vi "FPGA Personality.vi"   [LabVIEW 2020]
uses:
  <vilib>/rvi/Emulation/niFpgaGetClockAttributes.vi
  <vilib>/rvi/Emulation/niFpgaSctlEmulationGetInTimedLoop.vi
  <vilib>/rvi/Emulation/niFpgaEmulationReportErrorSimple.vi
  <vilib>/rvi/Emulation/niFpgaCriticalErrorInLSC.vi
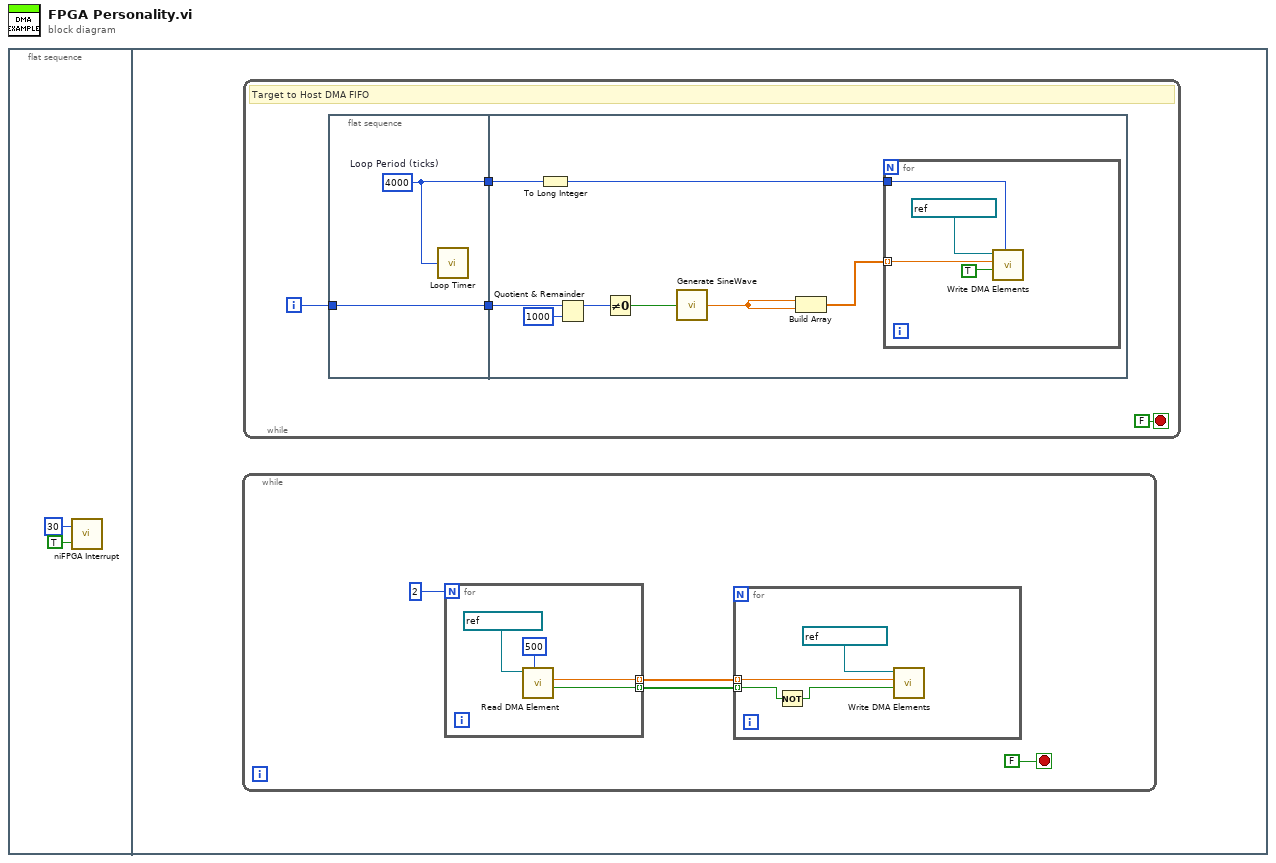
[diagram p0: block diagram]
diagram:
  n1 = flat-sequence {
    frame #0 {
      n2 = call <vilib>:"niFPGA Interrupt.vi"("Wait Until Cleared (F)"=TRUE, "IRQ Number (0)"=u8 30) -> ()  [unwired: 1 in]
    }
    frame #1 {
      n3 = while {
        stop <- FALSE stop-if-true
        n4 = for {
          N: 2 -> [_]
          tunnel: [w12] -> w4 mode=indexing
          tunnel: [w11] -> w3 mode=indexing
          n5 = call "Read DMA Element.vi"("Timeout"=500, "DMA Refnum in"=refnum<k21> "Incoming" ("FIFO In")) -> ("isTimeout ?"=w11:bool, "DMA Element"=w12:sgl)  [unwired: 7 in, 1 out]
        }
        n6 = for {
          tunnel: w4 -> [w8] mode=indexing
          tunnel: w3 -> [w7] mode=indexing
          n7 = Not(x=w7) -> (.not. x?=w9:bool)
          n8 = call "Write DMA Elements.vi"("isValid ?"=w9, "DMA Element"=w8, "FIFO Refnum in"=refnum<k21> "Outgoing2" ("FIFO In")) -> ()  [unwired: 8 in, 1 out]
        }
      }
      n9 = while {
        i -> [w16]
        stop <- FALSE stop-if-true
        # "Target to Host DMA FIFO"
        n10 = flat-sequence {
          tunnel: [w20] -> w18
          tunnel: w16 -> [w19]
          tunnel: [w19] -> w15
          tunnel: w18 -> [w28]
          tunnel: w15 -> [w24]
          frame #0 {
            w20 = u32 4000  # Loop Period (ticks)
            n11 = call "Loop Timer"("Count(Ticks)"=w20) -> ()  [unwired: 1 out]
          }
          frame #1 {
            n12 = To Long Integer(number=w28) -> (32bit integer=w27:i32)
            n13 = Quotient & Remainder(x=w24, y=1000) -> (x-y*floor(x/y)=w22:i32)  [unwired: 1 out]
            n14 = Not Equal To 0?(x=w22) -> (x != 0?=w21:bool)
            n15 = call "Generate SineWave.vi"("GenSine"=w21) -> ("Sine Point"=w25:sgl)
            n16 = Build Array(w25, w25) -> (w26:sgl[])
            n17 = for {
              tunnel: w27 -> [w30]
              tunnel: w26 -> [w29] mode=indexing
              n18 = call "Write DMA Elements.vi"("Timeout"=w30, "isValid ?"=TRUE, "DMA Element"=w29, "FIFO Refnum in"=refnum<k21> "Outgoing1" ("FIFO In")) -> ()  [unwired: 7 in, 1 out]
            }
          }
        }
      }
    }
  }
